vi "Midbrain Main.vi"(10 "Waypoint Queue Ref":T1, 11 "Notifier Ref":T2) -> ()   [LabVIEW 2013]
uses:
  Data/TypeDefs/Notifiers.ctl
  Data/TypeDefs/UTM Location.ctl
  Data/TypeDefs/Sail Set Suggestions.ctl
  Data/TypeDefs/Rudder Set Suggestions.ctl
  Data/TypeDefs/OverrideInformation.ctl
  Data/TypeDefs/OverrideMode.ctl
  Data/TypeDefs/MotorSetup.ctl
  Data/TypeDefs/DynamixelSetupInfo.ctl
  Data/TypeDefs/AirmarStatus.ctl
  Data/TypeDefs/HardwareOnline.ctl
  Data/TypeDefs/DynamixelCycleTracker.ctl
  Data/TypeDefs/RC Input Values.ctl
  Classes/Waypoint/Waypoint.lvclass
  Data/TypeDefs/Queues.ctl
panel:
  out "MidBrain Act Loop Counter":i32
  out "MidBrain Sense Loop Counter":i32
  out "Midbrain Think Loop Counter":i32
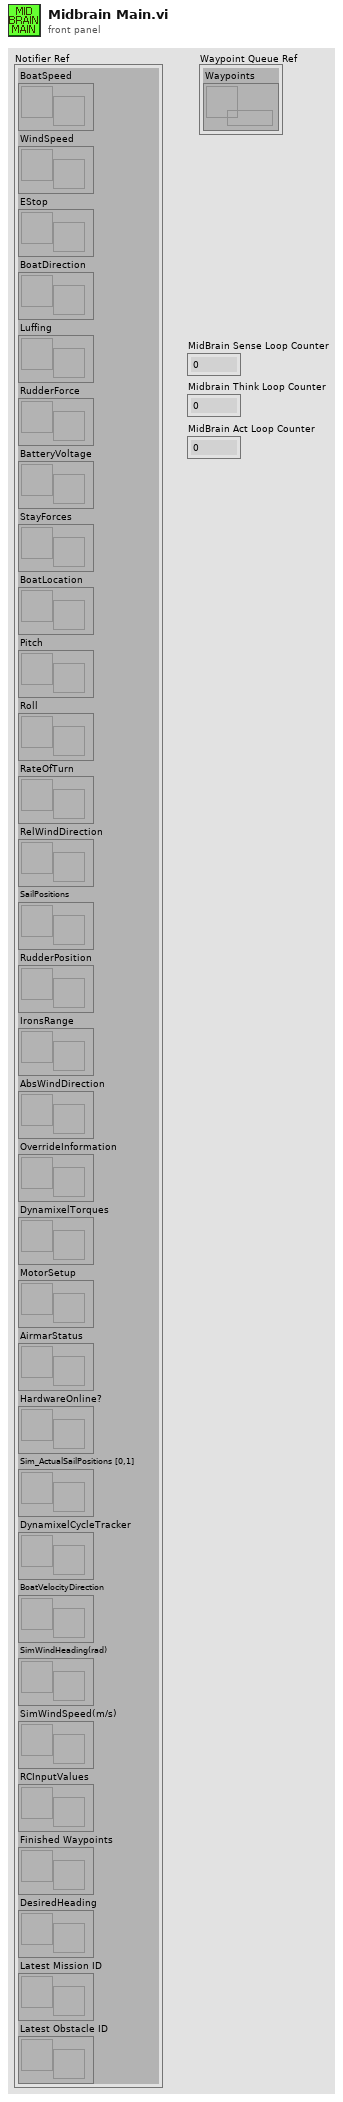
[diagram p1: front panel]
types:
  T1 = typedef "Queues.ctl" = cluster{"Waypoints":refnum<queue>}
  T2 = typedef "Notifiers.ctl" = cluster{"BoatSpeed":refnum<notifier>, "WindSpeed":refnum<notifier>, "EStop":refnum<notifier>, "BoatDirection":refnum<notifier>, "Luffing":refnum<notifier>, "RudderForce":refnum<notifier>, "BatteryVoltage":refnum<notifier>, "StayForces":refnum<notifier>, "BoatLocation":refnum<notifier>, "Pitch":refnum<notifier>, "Roll":refnum<notifier>, "RateOfTurn":refnum<notifier>, "RelWindDirection":refnum<notifier>, "SailPositions":refnum<notifier>, "RudderPosition":refnum<notifier>, "IronsRange":refnum<notifier>, "AbsWindDirection":refnum<notifier>, "OverrideInformation":refnum<notifier>, "DynamixelTorques":refnum<notifier>, "MotorSetup":refnum<notifier>, "AirmarStatus":refnum<notifier>, "HardwareOnline?":refnum<notifier>, "Sim_ActualSailPositions [0,1]":refnum<notifier>, "DynamixelCycleTracker":refnum<notifier>, "BoatVelocityDirection":refnum<notifier>, "SimWindHeading(rad)":refnum<notifier>, "SimWindSpeed(m/s)":refnum<notifier>, "RCInputValues":refnum<notifier>, "Finished Waypoints":refnum<notifier>, "DesiredHeading":refnum<notifier>, "Latest Mission ID":refnum<notifier>, "Latest Obstacle ID":refnum<notifier>}
  T3 = typedef "Boat Regimes.ctl" = cluster{"Sailing Regime":T4, "Emergency Regimes":T5, "Emergency?":bool, "CCW?":bool, "Force direction?":bool}
  T4 = typedef "Sailing Regimes.ctl" = enum16{"Tack - Bow across wind", "Upwind - Starboard Tack", "Turn between Upwind/Reach - Starboard Tack", "Reach - Starboard Tack", "Turn between Reach/Run - Starboard Tack", "Run - Starboard Tack", "Jibe - Stern across wind", "Run - Port Tack", "Turn between Reach/Run - Port Tack", "Reach - Port Tack", "Turn between Upwind/Reach - Port Tack", "Upwind - Port Tack"}
  T5 = typedef "Emergency Regimes.ctl" = enum16{"NO EMERGENCY", "No Knockdown", "Obstacle Avoid"}
  T6 = typedef "Rudder Set Suggestions.ctl" = dbl
  T7 = typedef "Sail Set Suggestions.ctl" = cluster{"MainSailSuggestion":dbl, "JibSailSuggestion":dbl}
  T8 = typedef "HardwareOnline.ctl" = cluster{"AirmarOnline":bool, "WindvaneOnline":bool, "HemisphereOnline":bool, "StayForceOnline":bool, "BatteryVoltageOnline":bool, "AccelerometerOnline":bool, "MainDynamixel Online":bool, "JibDynamixel Online":bool, "RudderDynamixel Online":bool}
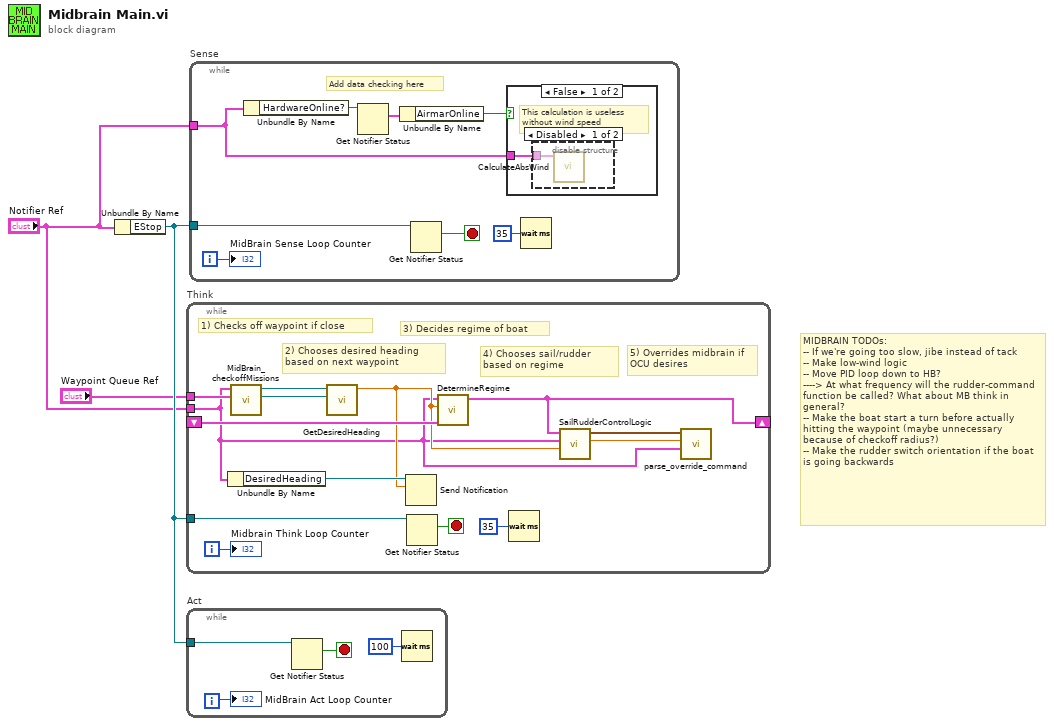
[diagram p0: block diagram]
diagram:
  # "MIDBRAIN TODOs:\n-- If we're going too slow, jibe instead of tack\n-- Make low-wind logic\n-- Move PID loop down to HB?\n----> At what frequency will the rudder-command function be called? What about MB think in general?\n-- Make the boat start a turn before actually hitting the waypoint (maybe unnecessary because of checkoff radius?)\n-- Make the rudder switch orientation if the boat is going backwards"
  n1 = Unbundle By Name("Notifier Ref") -> ("EStop"=w3:refnum<notifier>)
  n2 = while "Think" {
    tunnel: w3 -> [w17]
    shift-right: [w14] -> _
    shift-left: _ -> [w15]
    tunnel: "Notifier Ref" -> [w4]
    tunnel: "Waypoint Queue Ref" -> [w13]
    i -> [w10]
    stop <- w16 stop-if-true
    # "5) Overrides midbrain if OCU desires"
    # "4) Chooses sail/rudder based on regime"
    # "3) Decides regime of boat"
    # "2) Chooses desired heading based on next waypoint"
    # "1) Checks off waypoint if close"
    n3 = Unbundle By Name(w4) -> ("DesiredHeading"=w6:refnum<notifier>)
    n4 = call "MidBrain_checkoffMissions.vi"("Mission QueueRef"=w13, "NotifierReff"=w4) -> ("Waypoints Queue Out"=w11:refnum<queue>, "BoatLocation Notifier Out"=w12:refnum<notifier>)  [unwired: 8 in]
    n5 = call "GetDesiredHeading.vi"("Waypoints"=w11, "BoatLocation"=w12) -> ("Desired Heading"=w5:dbl)  [unwired: 9 in]
    n6 = Send Notification(notification=w5, notifier=w6) -> ()  [unwired: 1 in, 2 out]
    n7 = Get Notifier Status(notifier=w17) -> (current notification=w16:bool)  [unwired: 1 in, 4 out]
    n8 = call "DetermineRegime.vi"("Last Commanded Boat Regime"=w15, "Desired Heading (deg)"=w5, "NotifierReff"=w4) -> ("Commanded Boat Regime"=w14:T3)  [unwired: 8 in]
    n9 = Wait (ms)(milliseconds to wait=u32 35) -> ()  [unwired: 1 out]
    n10 = call "SailRudderControlLogic.vi"("DesiredHeading"=w5, "NotifierReff"=w4, "Commanded Boat Regime"=w14) -> ("Suggested Rudder Setpoint"=w7:T6, "Suggested Sail Setpoints"=w8:T7)  [unwired: 7 in]
    n11 = call "parse_override_command.vi"("Notifier Ref."=w4, "Midbrain Rudder Setpoint"=w7, "Midbrain Sail Setpoints"=w8) -> ()  [unwired: 9 in]
    "Midbrain Think Loop Counter" <- w10
  }
  n12 = while "Act" {
    tunnel: w3 -> [w21]
    i -> [w19]
    stop <- w20 stop-if-true
    n13 = Get Notifier Status(notifier=w21) -> (current notification=w20:bool)  [unwired: 1 in, 4 out]
    n14 = Wait (ms)(milliseconds to wait=u32 100) -> ()  [unwired: 1 out]
    "MidBrain Act Loop Counter" <- w19
  }
  n15 = while "Sense" {
    tunnel: w3 -> [w29]
    tunnel: "Notifier Ref" -> [w27]
    i -> [w23]
    stop <- w28 stop-if-true
    # "Add data checking here"
    n16 = Unbundle By Name(w27) -> ("HardwareOnline?"=w26:refnum<notifier>)
    n17 = Get Notifier Status(notifier=w26) -> (current notification=w25:T8)  [unwired: 1 in, 4 out]
    n18 = Unbundle By Name(w25) -> ("AirmarOnline"=w24:bool)
    n19 = Get Notifier Status(notifier=w29) -> (current notification=w28:bool)  [unwired: 1 in, 4 out]
    n20 = case shown="False" w24 {
      tunnel: w27 -> [w30 _]
      frame False {
        # "This calculation is useless without wind speed"
        n21 = disable-structure shown="Disabled" {
          disable-tunnel: w30 -> [w31 _]
          frame Disabled {
            n22 = call "CalculateAbsWind.vi"("NotifierReff"=w31) -> ()  [unwired: 11 in]
          }
          frame Enabled {
          }
        }
      }
      frame True {
      }
    }
    n23 = Wait (ms)(milliseconds to wait=u32 35) -> ()  [unwired: 1 out]
    "MidBrain Sense Loop Counter" <- w23
  }
